vi "Open_HDF5.vi"() -> ()   [LabVIEW 2018]
uses:
  <vilib>/addons/h5labview2/base/h5o_type.ctl
  HDF5/TC_Data_Structure.ctl
  HDF5/lib_path_mod_20200519.vi
  <vilib>/addons/h5labview2/base/H5Equery.vi
  <vilib>/addons/h5labview2/dataset/H5Dread.llb/H5Dread.xnode
  <vilib>/addons/h5labview2/file/H5F.lvlib
  <vilib>/addons/h5labview2/group/H5G.lvlib
  <vilib>/addons/h5labview2/dataset/H5D.lvlib
  <vilib>/addons/h5labview2/attrib/H5Aread.llb/H5Aread.xnode
  <vilib>/addons/h5labview2/attrib/H5A.lvlib
panel:
  out "attribs":string[](array[string])
  out "found? 2":bool
  out "data 2":variant
  out "data 3":T1[][](array[typedef])
  out "found?":bool
  out "types":T2[](array[typedef])
  out "data":variant
  out "names":string[](array[string])
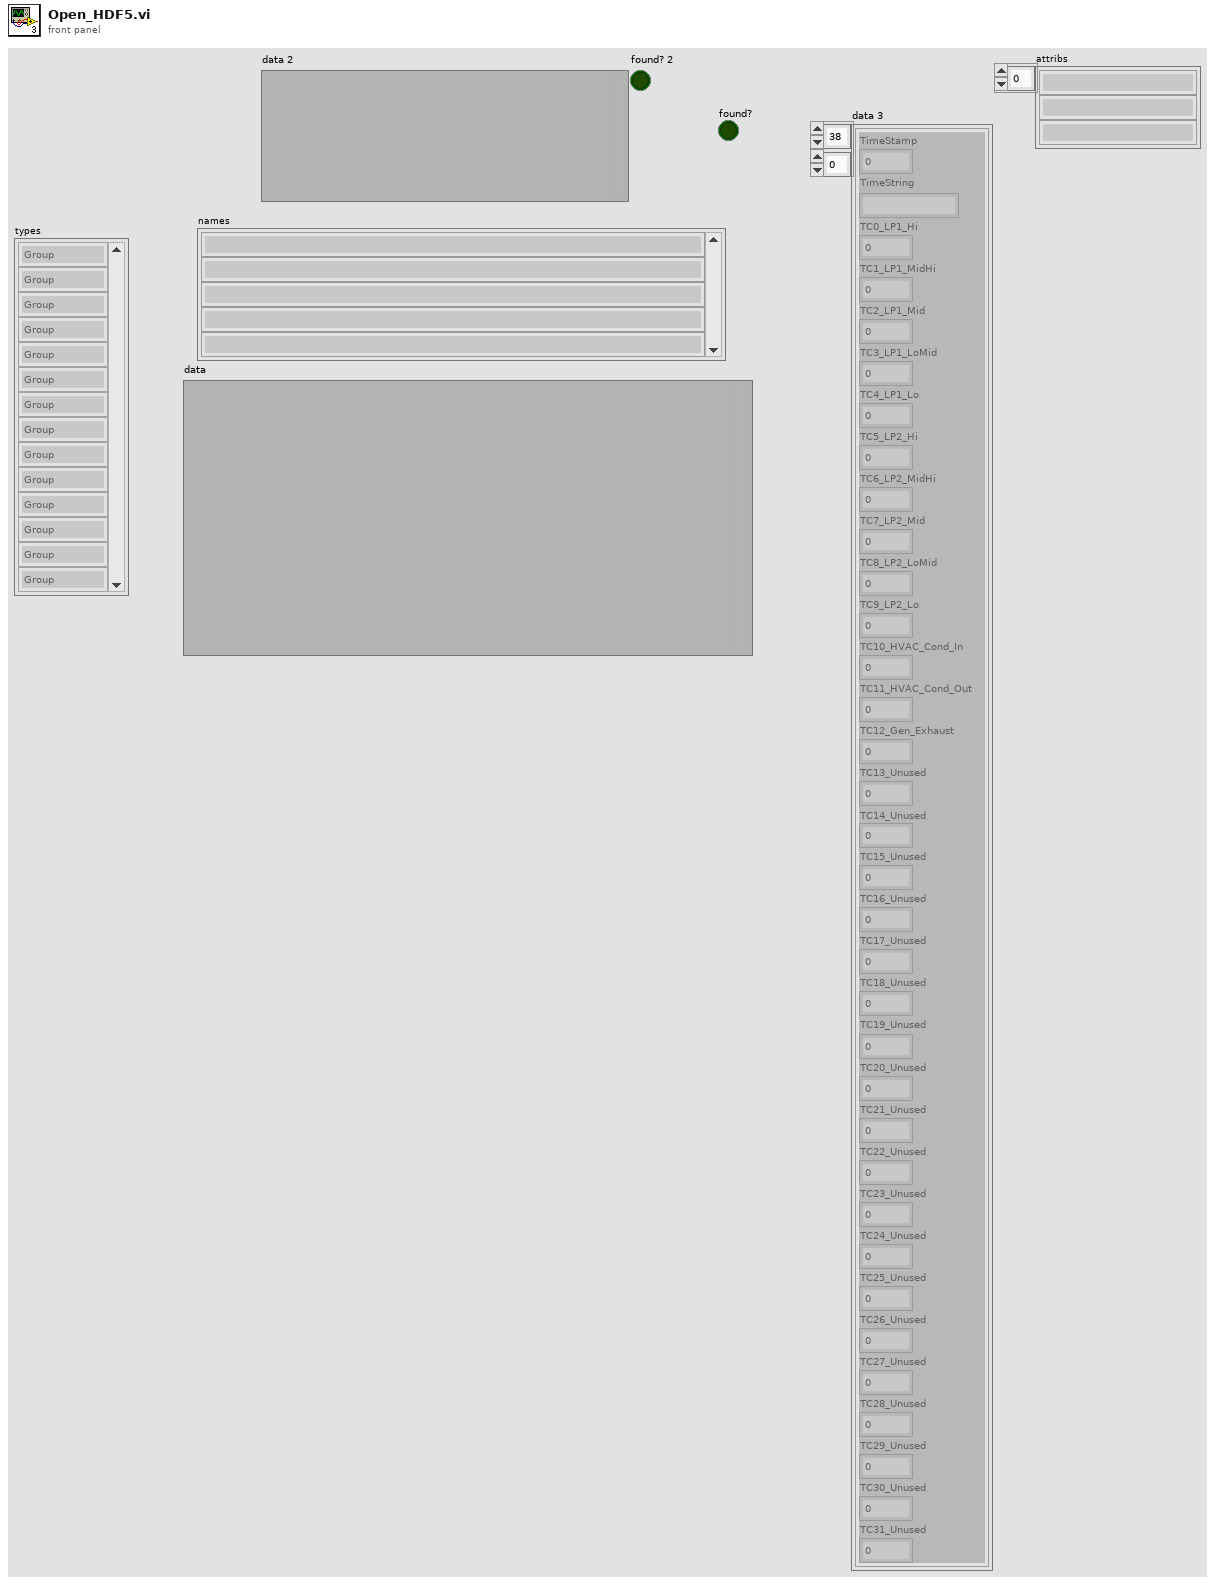
[diagram p1: front panel]
types:
  T1 = typedef "TC_Data_Structure.ctl" = cluster{"TimeStamp":dbl, "TimeString":string, "TC0_LP1_Hi":dbl, "TC1_LP1_MidHi":dbl, "TC2_LP1_Mid":dbl, "TC3_LP1_LoMid":dbl, "TC4_LP1_Lo":dbl, "TC5_LP2_Hi":dbl, "TC6_LP2_MidHi":dbl, "TC7_LP2_Mid":dbl, "TC8_LP2_LoMid":dbl, "TC9_LP2_Lo":dbl, "TC10_HVAC_Cond_In":dbl, "TC11_HVAC_Cond_Out":dbl, "TC12_Gen_Exhaust":dbl, "TC13_Unused":dbl, "TC14_Unused":dbl, "TC15_Unused":dbl, "TC16_Unused":dbl, "TC17_Unused":dbl, "TC18_Unused":dbl, "TC19_Unused":dbl, "TC20_Unused":dbl, "TC21_Unused":dbl, "TC22_Unused":dbl, "TC23_Unused":dbl, "TC24_Unused":dbl, "TC25_Unused":dbl, "TC26_Unused":dbl, "TC27_Unused":dbl, "TC28_Unused":dbl, "TC29_Unused":dbl, "TC30_Unused":dbl, "TC31_Unused":dbl}
  T2 = typedef "h5o_type.ctl" = enum8{"Group", "Dataset", "Named type"}
  T3 = typedef "hid_t.ctl" = i32
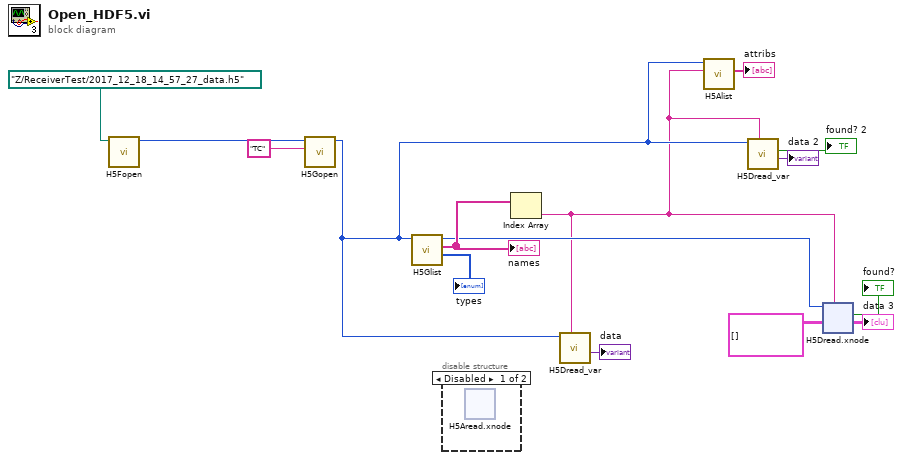
[diagram p0: block diagram]
diagram:
  n1 = call <vilib>:"H5Fopen.vi"("path"=path "Z:/ReceiverTest/2017_12_18_14_57_27_data.h5") -> ("ref out"=w14:T3)  [unwired: 9 in, 1 out]
  n2 = call <vilib>:"H5Gopen.vi"("name"="TC", "ref in"=w14) -> ("group out"=w3:T3)  [unwired: 8 in, 1 out]
  n3 = call <vilib>:"H5Glist.vi"("ref in"=w3) -> ("types"=→"types":T2[], "names"=w13:string[], "ref out"=w5:T3)  [unwired: 7 in, 1 out]
  "names" <- w13
  n4 = disable-structure shown="Disabled" {
    frame Disabled {
      n5 = xnode "H5Aread.xnode"() -> ()  [unwired: 6 in, 4 out]
    }
    frame Enabled {
    }
  }
  n6 = Index Array(array=w13) -> (element=w2:string)  [unwired: 1 in]
  n7 = call <vilib>:"H5Dread_var.vi"("dataset name (this)"=w2, "ref in"=w3) -> ("data"=→"data":variant)  [unwired: 6 in, 3 out]
  n8 = call <vilib>:"H5Alist.vi"("object (.)"=w2, "ref in"=w3) -> ("attribs"=→"attribs":string[])  [unwired: 7 in, 2 out]
  n9 = call <vilib>:"H5Dread_var.vi"("dataset name (this)"=w2, "ref in"=w3) -> ("data"=→"data 2":variant, "found?"=→"found? 2":bool)  [unwired: 6 in, 2 out]
  n10 = xnode "H5Dread.xnode"("dataset name (this)"=w2, "default"=T1[][] [] ("Array"), "ref in"=w5) -> ("data"=→"data 3":T1[][], "found?"=→"found?":bool)  [unwired: 3 in, 2 out]
